vi "main.vi"() -> ()   [LabVIEW 2016]
uses:
  TypeDefs/details.ctl
  TypeDefs/settings.ctl
  TypeDefs/State Enumerate Ring.ctl
  <vilib>/Utility/file.llb/Write Delimited Spreadsheet (DBL).vi
  <instrlib>/Keithley 24XX/Public/Data/Read (Multiple Points).vi
  <instrlib>/Keithley 24XX/Keithley 24XX.lvlib
panel:
  out "Data Output Folder":path
  out "Settings folder path":path
  out "Date array":string[](array[string])
  out "Abort initalisation?":bool
  in  "Tab Control":enum32{"Setup", "Advanced"}(tab)
  in  "Scan settings":T1={"Start voltage (V)"=0.0, "End voltage (V)"=10.0, "Number of steps"=11, "Measurement delay (ms)"=100.0, "Dual sweep"=1, "Stabilisation time (s)"=120.0, "Stabilisation mode"=0, "Stabilisation value (V or A) "=-5.0, "No. of repeat scans"=2.0, "Repeat scans"=0, "Logarithmic sweep"=1, "Electrode configuration"=0} {"Electrode configuration" items=["2-wire", "4-wire"]; "Logarithmic sweep" items=["False", "True"]; "Repeat scans" items=["False", "True"]; "No. of repeat scans" min=1.0 step=1.0; "Stabilisation mode" items=["V", "I"]; "Dual sweep" items=["False", "True"]; "Measurement delay (ms)" min=0.0}
  out "Keithley 2400":bool
  in  "User Name":string
  in  "Exeriment Title":string
  out "Status:":string
  in  "Device details":T2={"Cell Label"="", "Area (cm^2)"=0.0919, "Notes"="", "Scan settings"=0} {"Scan settings" items=["Default", "S01-F-0.1-200-67-0.01-120_-5", "S02-S-0.1-200-67-10-120_-5", "S03-F-0.1-200-67-0.01-0_0", "S04-S-0.1-200-67-10-0_0", "S05-F-0.1-200-67-0.01-10_-5", "S06-F-0.1-200-65-0.01-120_-5", "S07-F-0.001-200-67-0.01-120_-5", "S08-F-0.001-200-67-0.01-120_-10", "S09-F-0.001-200-67-0.01-120_-2", "S12-F-0.1-200-67-0.05-0-0", "S13-F-0.1-200-67-0.01-0-0", "S14-F-0.1-200-67-0.1-0-0", "S15-F-0.01-200-67-0.01-0-0", "S16-F-0.01-20-67-0.01-0-0", "S17-F-0.01-20-67-0.1-0-0", "S18-F-0.1-200-67-0.01-120_-1", "S19-F-0.1-200-67-0.01-120_-1.5", "S20-F-0.1-200-67-0.01-120_-2", "S21-F-0.1-200-67-0.01-120_-2.5", "S22-F-0.1-200-67-0.1-120_-1", "S23-F-0.1-200-67-0.1-120_-2", "S24-F-0.1-200-67-0.1-120_-5", "S25-F-0.1-200-67-0.1-120_-10", "S26-F-0.1-200-67-0.01-120_-10", "S27-F-0.1-200-67-0.01-120_-15", "S28-F-0.1-200-67-0.1-120_-15", "S29-F-0.1-200-67-0.01-12_-5", "S30-F-0.1-200-67-0.01-0-0", "S31-S-0.1-200-67-1-30_-1", "S32-F-0.1-200-200-0.01-120_-1", "S33-F-0.1-200-200-0.01-120_-5", "S34-F-0.1-200-67-0-0_0", "S35-F-0.1-200-67-0-120_-1", "S36-F-0.1-200-67-0-120_-5", "S37-F-0.1-50-67-0.01-0_0", "S38-F-0.1-50-67-0.01-120_1", "S39-F-0.1-100-0.01-120_5", "S40-F-0.1-100-0.002-120-10", "S41-F-0.1-200-0.002-120-10", "S42-F-0.1-200-0.01-120-10", "S43-F-0.1-20-0.01-0_0", "S44-F-0.1-20-67-2-0_0", "S45-F-0.1-80-67-2-0_0", "S46-F-0.1-80-67-2-120_-1"]}
  in  "Delete settings":bool
  in  "Save new settings":bool
  in  "Check Saved Settings":u16(ring) items=["Default", "S01-F-0.1-200-67-0.01-120_-5", "S02-S-0.1-200-67-10-120_-5", "S03-F-0.1-200-67-0.01-0_0", "S04-S-0.1-200-67-10-0_0", "S05-F-0.1-200-67-0.01-10_-5", "S06-F-0.1-200-65-0.01-120_-5", "S07-F-0.001-200-67-0.01-120_-5", "S08-F-0.001-200-67-0.01-120_-10", "S09-F-0.001-200-67-0.01-120_-2", "S12-F-0.1-200-67-0.05-0-0", "S13-F-0.1-200-67-0.01-0-0", "S14-F-0.1-200-67-0.1-0-0", "S15-F-0.01-200-67-0.01-0-0", "S16-F-0.01-20-67-0.01-0-0", "S17-F-0.01-20-67-0.1-0-0", "S18-F-0.1-200-67-0.01-120_-1", "S19-F-0.1-200-67-0.01-120_-1.5", "S20-F-0.1-200-67-0.01-120_-2", "S21-F-0.1-200-67-0.01-120_-2.5", "S22-F-0.1-200-67-0.1-120_-1", "S23-F-0.1-200-67-0.1-120_-2", "S24-F-0.1-200-67-0.1-120_-5", "S25-F-0.1-200-67-0.1-120_-10", "S26-F-0.1-200-67-0.01-120_-10", "S27-F-0.1-200-67-0.01-120_-15", "S28-F-0.1-200-67-0.1-120_-15", "S29-F-0.1-200-67-0.01-12_-5", "S30-F-0.1-200-67-0.01-0-0", "S31-S-0.1-200-67-1-30_-1", "S32-F-0.1-200-200-0.01-120_-1", "S33-F-0.1-200-200-0.01-120_-5", "S34-F-0.1-200-67-0-0_0", "S35-F-0.1-200-67-0-120_-1", "S36-F-0.1-200-67-0-120_-5", "S37-F-0.1-50-67-0.01-0_0", "S38-F-0.1-50-67-0.01-120_1", "S39-F-0.1-100-0.01-120_5", "S40-F-0.1-100-0.002-120-10", "S41-F-0.1-200-0.002-120-10", "S42-F-0.1-200-0.01-120-10", "S43-F-0.1-20-0.01-0_0", "S44-F-0.1-20-67-2-0_0", "S45-F-0.1-80-67-2-0_0", "S46-F-0.1-80-67-2-120_-1"]
  in  "Save New Settings As...":string
  in  "Update":bool
  in  "Exit":bool
  out "JV Curve":cluster{dbl[], dbl[]}(graph)
  in  "Start Scan":bool
  in  "error in (no error) 3":errorcluster
  in  "VISA resource name":refnum<visa-resource-name>="GPIB1::26::INSTR"
  # "Connected instruments"
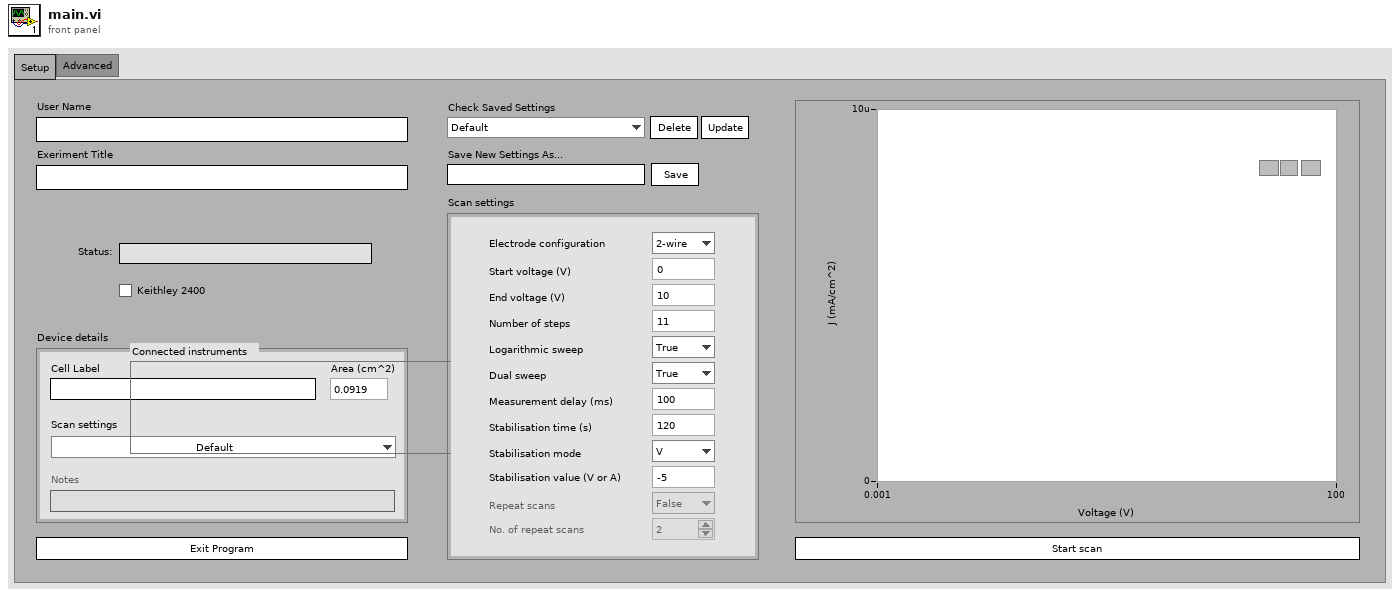
[diagram p1: front panel]
types:
  T1 = typedef "settings.ctl" = cluster{"Start voltage (V)":dbl, "End voltage (V)":dbl, "Number of steps":u32, "Measurement delay (ms)":dbl, "Dual sweep":u16, "Stabilisation time (s)":dbl, "Stabilisation mode":u16, "Stabilisation value (V or A) ":dbl, "No. of repeat scans":dbl, "Repeat scans":u16, "Logarithmic sweep":u16, "Electrode configuration":u16}
  T2 = typedef "details.ctl" = cluster{"Cell Label":string, "Area (cm^2)":dbl, "Notes":string, "Scan settings":u16}
  T3 = typedef "State Enumerate Ring.ctl" = enum16{"Initialise", "Idle", "Measure", "Notify"}
  T4 = enum8{"Enabled", "Disabled", "Disabled and Grayed Out"}
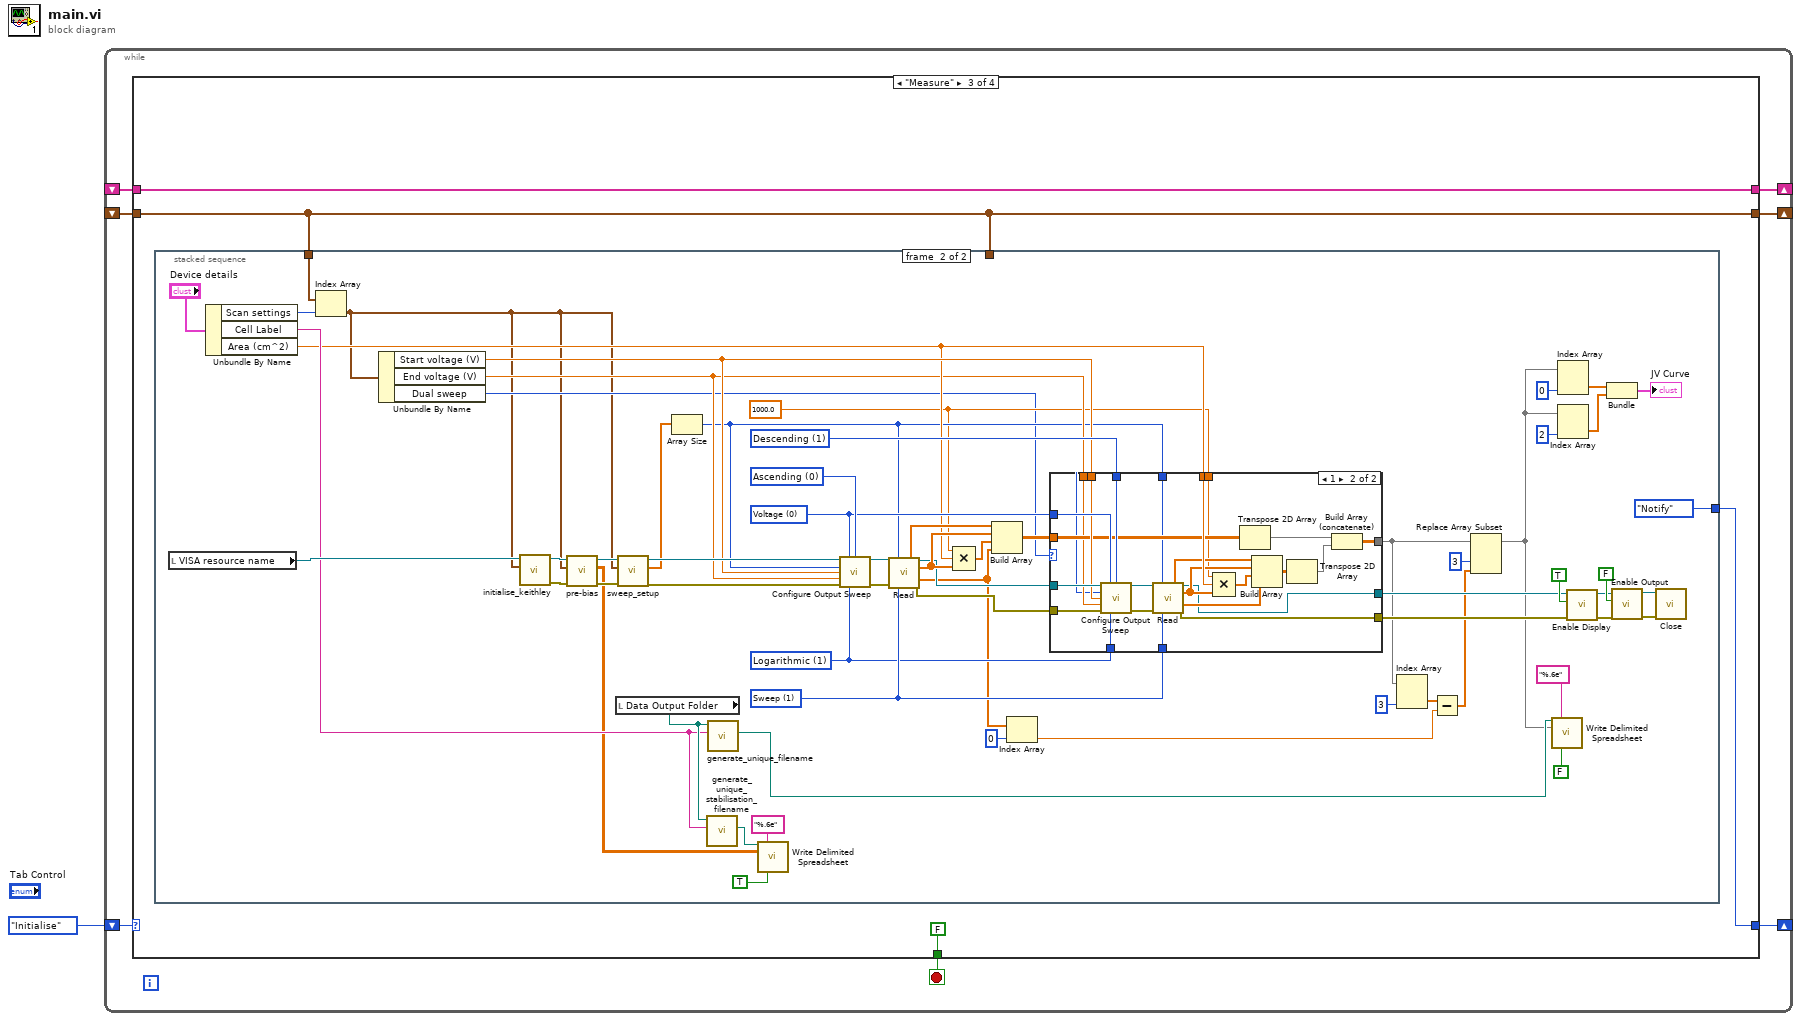
[diagram p0: block diagram]
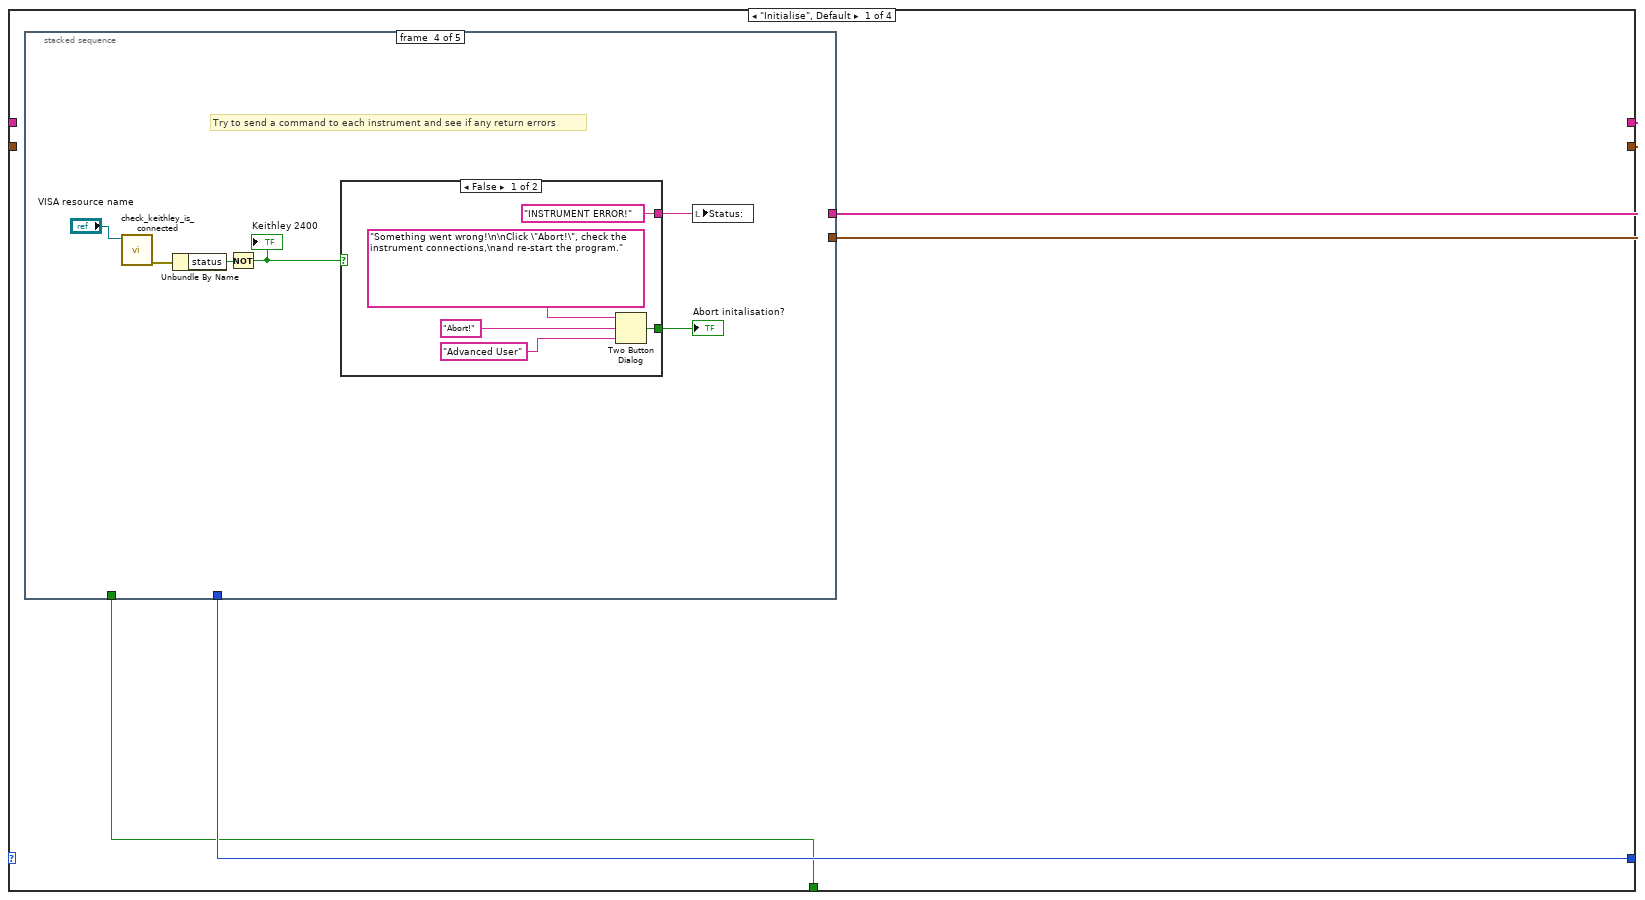
[diagram p2: hidden frame]
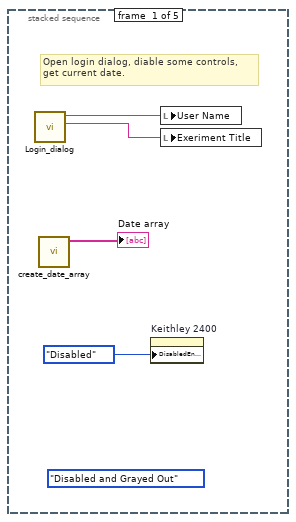
[diagram p3: hidden frame]
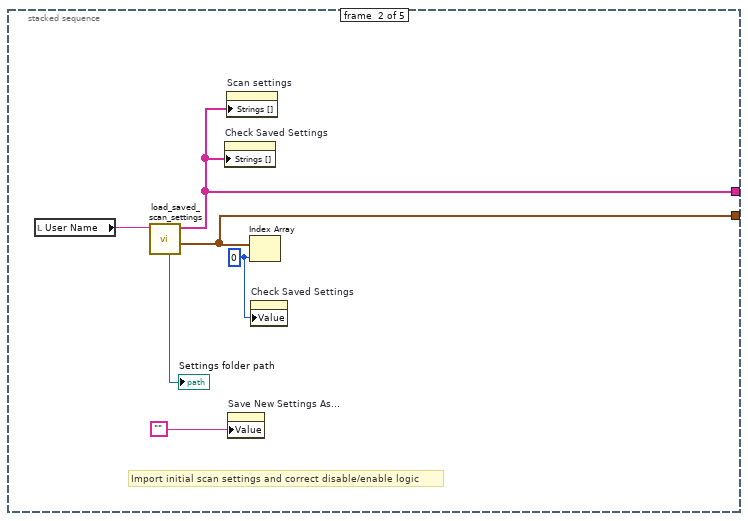
[diagram p4: hidden frame]
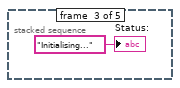
[diagram p5: hidden frame]
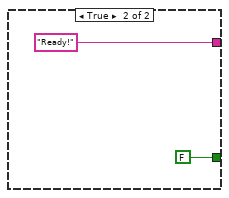
[diagram p6: hidden frame]
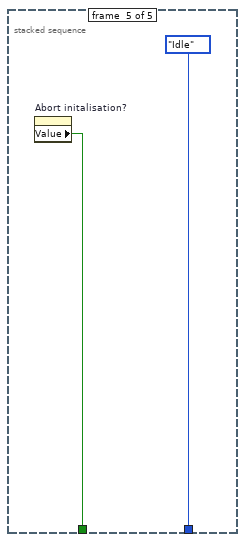
[diagram p7: hidden frame]
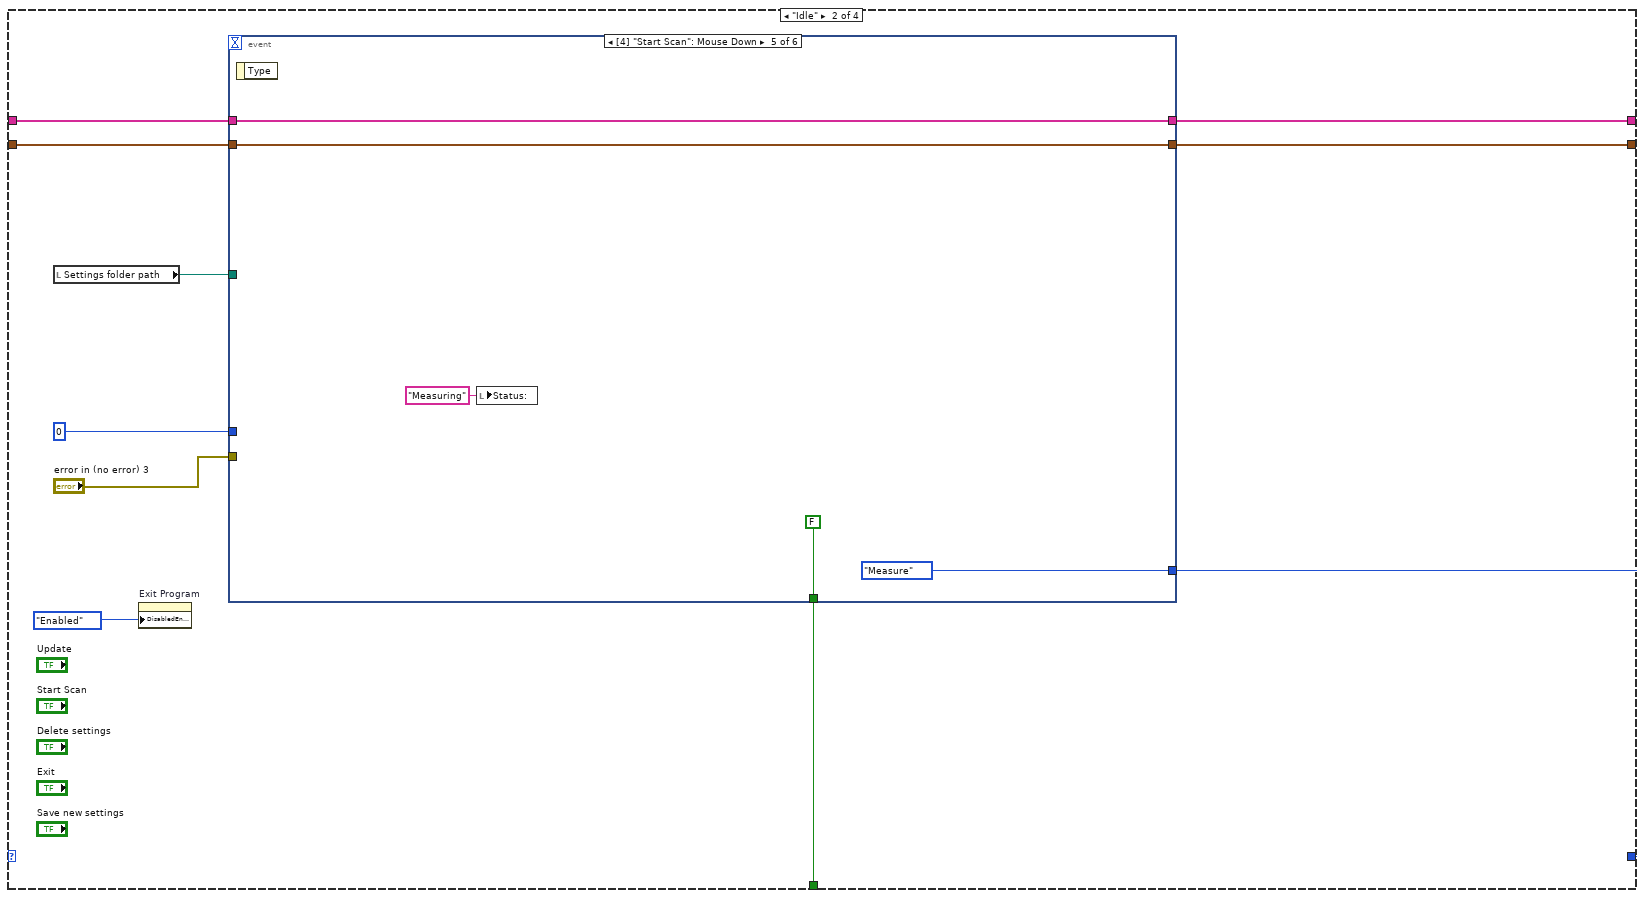
[diagram p8: hidden frame]
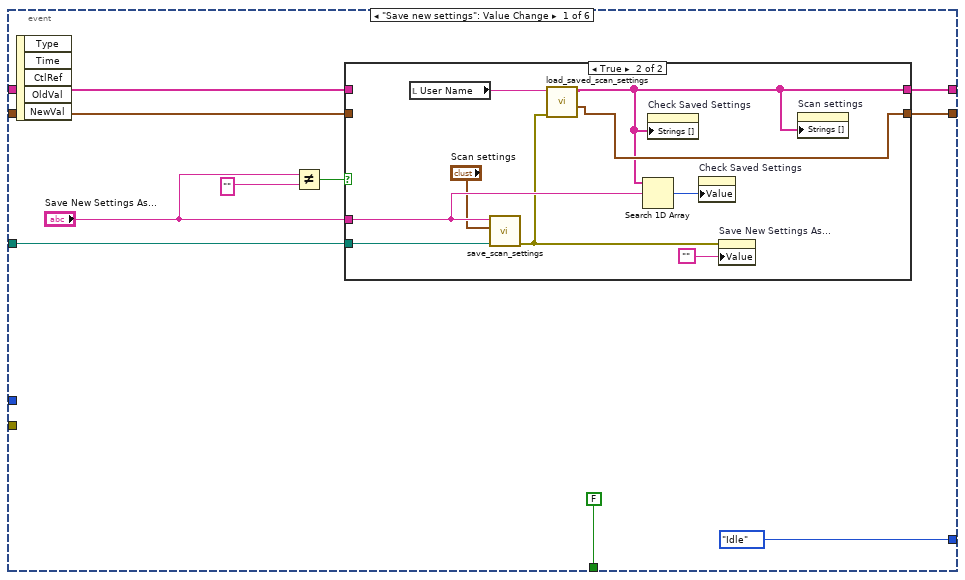
[diagram p9: hidden frame]
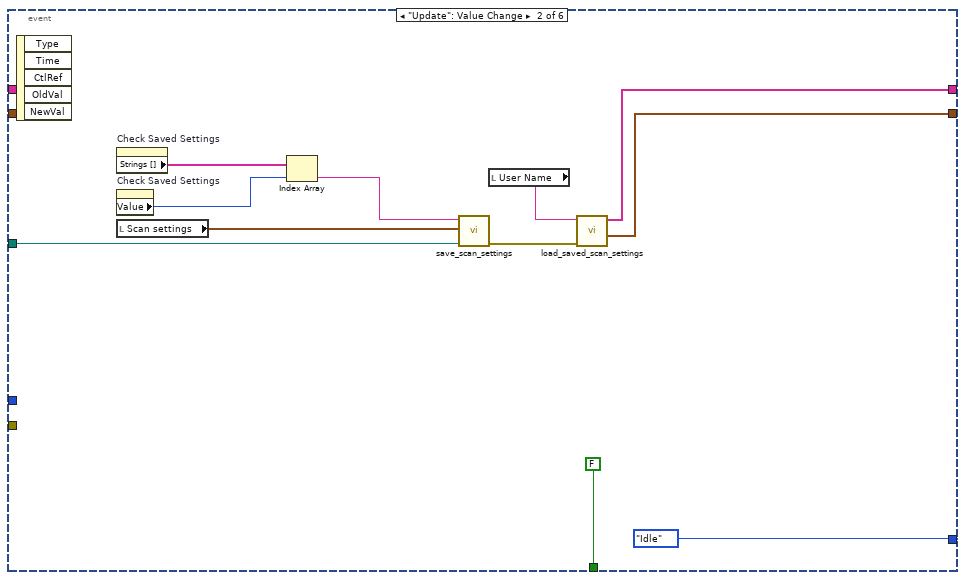
[diagram p11: hidden frame]
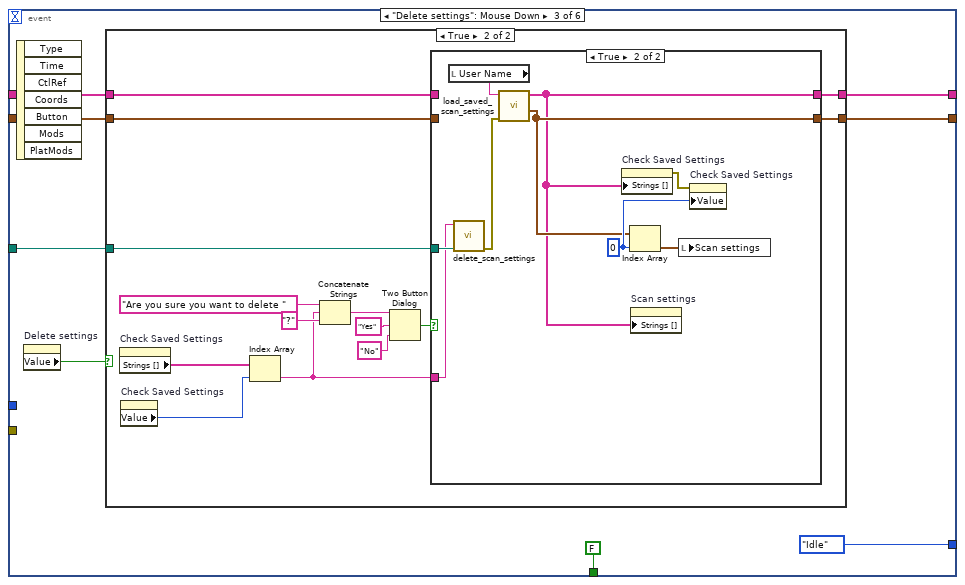
[diagram p12: hidden frame]
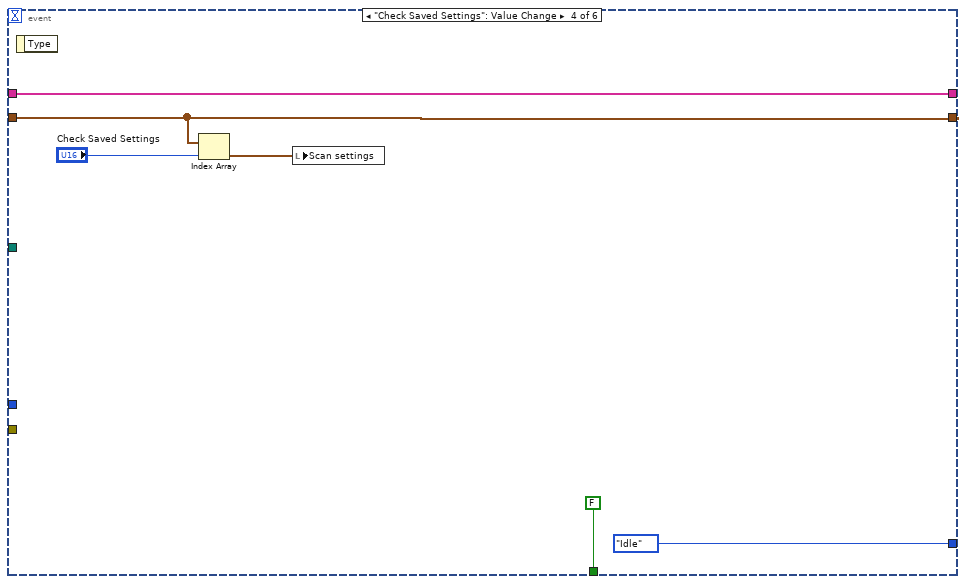
[diagram p15: hidden frame]
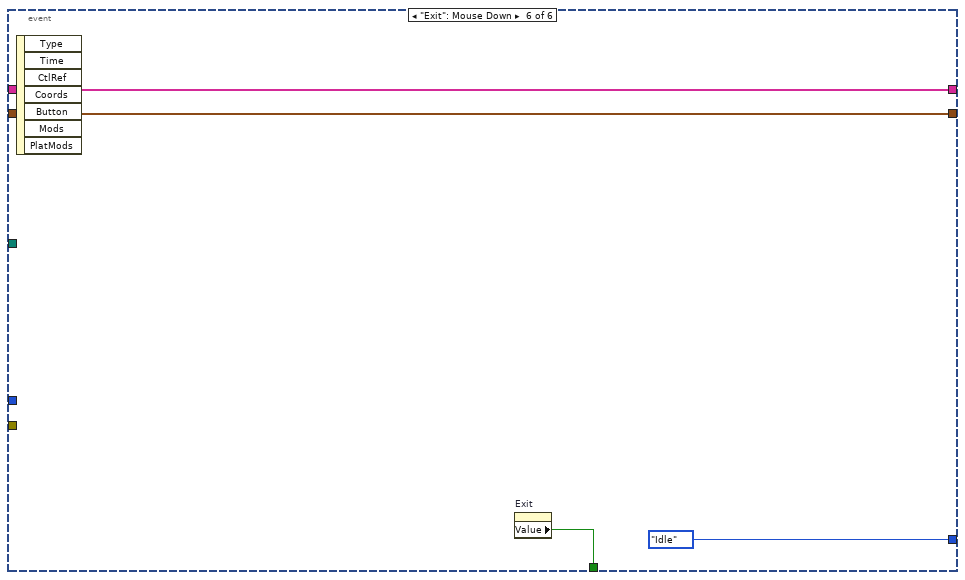
[diagram p16: hidden frame]
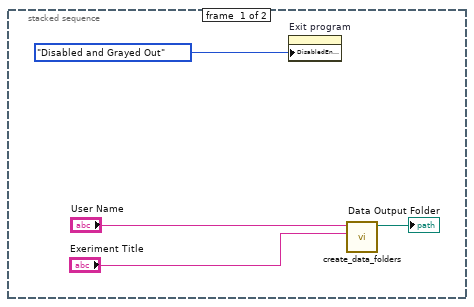
[diagram p17: hidden frame]
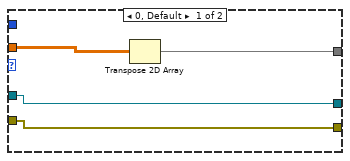
[diagram p18: hidden frame]
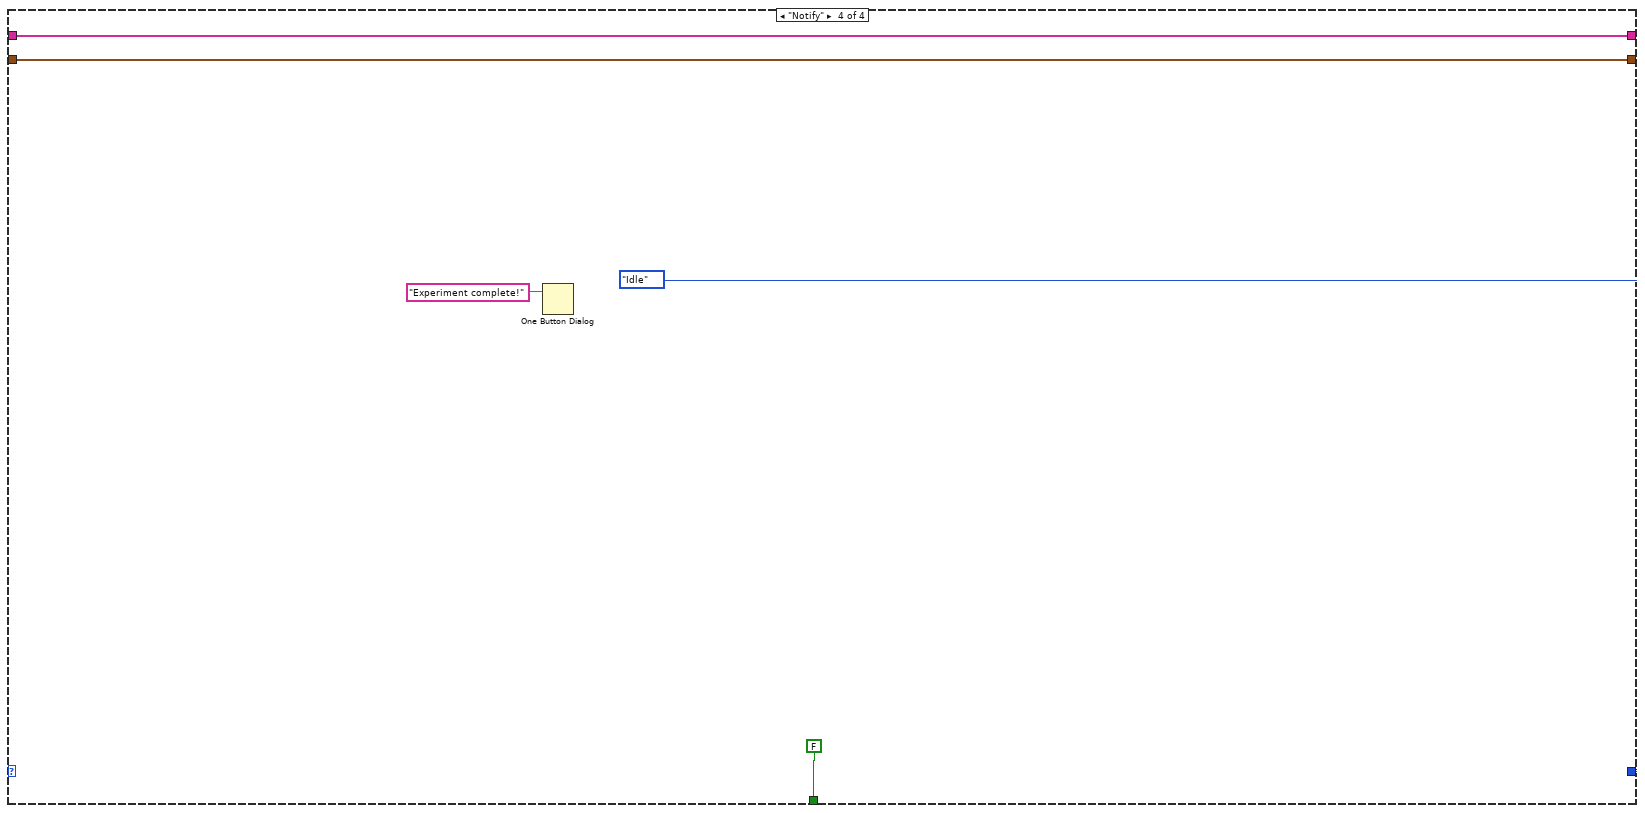
[diagram p19: hidden frame]
diagram:
  n1 = while {
    shift-right: [w3] -> _
    shift-left: _ -> [w5]
    shift-right: [w4] -> _
    shift-left: _ -> [w6]
    shift-right: [w7] -> _
    shift-left: State_Enumerate_Ring."Initialise" ("Enum") -> [w8]
    stop <- w2 stop-if-true
    n2 = case shown="\"Measure\"" w8 {
      tunnel: [w12 w42 w132 State_Enumerate_Ring."Idle" ("Enum")] -> w7
      tunnel: w6 -> [_ w46 w131 w234]
      tunnel: w5 -> [_ w45 w133 w233]
      tunnel: [w10 w44 w131 w234] -> w4
      tunnel: [w9 w43 w133 w233] -> w3
      tunnel: [w11 w40 FALSE ("Value") FALSE ("Value")] -> w2
      frame "Initialise", Default {
        n3 = stacked-sequence {
          tunnel: [_ _ _ _ State_Enumerate_Ring."Idle" ("Enum")] -> w12
          tunnel: [_ _ _ _ w37] -> w11
          tunnel: [_ w22 _ _ _] -> w10
          tunnel: [_ w21 _ _ _] -> w9
          frame #0 {
            (unwired) T4."Disabled and Grayed Out" ("Disabled")
            # "Open login dialog, diable some controls,\nget current date."
            n4 = call "Login_dialog.vi"() -> ("Experiment title out"=w13:string, "User name out"=w14:string)  [unwired: 10 in]
            n5 = call "create_date_array.vi"() -> ("Date Array"=→"Date array":string[])  [unwired: 11 in]
            n6 = property on="Keithley 2400" class="Bool (strict)"("DisabledEnum"=T4."Disabled" ("Disabled")) -> ()  [unwired: 2 in, 2 out]
            n7 = local write "User Name"(w14) -> ()
            n8 = local write "Exeriment Title"(w13) -> ()
          }
          frame #1 {
            w19 = 0 ("index")
            # "Import initial scan settings and correct disable/enable logic"
            n9 = local read "User Name"() -> (w17:string)
            n10 = call "load_saved_scan_settings.vi"("User name"=w17) -> ("Scan settings array"=w21:T1[], "Scan settings name array"=w22:string[], "Settings folder path"=→"Settings folder path":path)  [unwired: 7 in, 1 out]
            n11 = property on="Check Saved Settings" class="Ring (strict)"("Strings []"=w22) -> ()  [unwired: 2 in, 2 out]
            n12 = property on="Scan settings" class="Ring (strict)"("Strings []"=w22) -> ()  [unwired: 2 in, 2 out]
            n13 = property on="Save New Settings As..." class="Str"("Value"="") -> ()  [unwired: 2 in, 2 out]
            n14 = Index Array(array=w21, index=w19) -> ()  [unwired: 1 out]
            n15 = property on="Check Saved Settings" class="Ring (strict)"("Value"=w19) -> ()  [unwired: 2 in, 2 out]
          }
          frame #2 {
            "Status:" <- "Initialising..." ("Instrument status")
          }
          frame #3 {
            # "Try to send a command to each instrument and see if any return errors"
            n16 = call "check_keithley_is_connected.vi"("VISA resource name"="VISA resource name") -> ("error out"=w29:errorcluster)  [unwired: 10 in]
            n17 = Unbundle By Name(w29) -> ("status"=w27:bool)
            n18 = Not(x=w27) -> (.not. x?=w25:bool)
            "Keithley 2400" <- w25
            n19 = case shown="False" w25 {
              tunnel: ["INSTRUMENT ERROR!" ("Instrument status") "Ready!" ("Instrument status")] -> w28
              tunnel: [w32 FALSE ("T button?")] -> w26
              frame False {
                n20 = Two Button Dialog(message="Something went wrong!\n\nClick \"Abort!\", check the instrument connections,\nand re-start the program.", 1:"Advanced User" ("T button name (\"OK\")"), 2:"Abort!" ("F button name (\"Cancel\")")) -> (T button?=w32:bool)
              }
              frame True {
              }
            }
            "Abort initalisation?" <- w26
            n21 = local write "Status:"(w28) -> ()
          }
          frame #4 {
            n22 = property on="Abort initalisation?" class="Bool (strict)"() -> ("Value"=w37:bool)  [unwired: 2 in, 2 out]
          }
        }
      }
      frame "Idle" {
        n23 = local read "Settings folder path"() -> (w39:path)
        n24 = property on="Exit Program" class="Bool (strict)"("DisabledEnum"=T4."Enabled" ("Disabled")) -> ()  [unwired: 2 in, 2 out]
        n25 = event shown="[4] \"Start Scan\": Mouse Down" {
          selector: _ -> [_ _ _ _ _ _]
          dyn-events: _ -> [_ _ _ _ _ _]
          timeout: _ -> [_ _ _ _ _ _]
          tunnel: 0 -> [_ _ _ _ _ _]
          tunnel: "error in (no error) 3" -> [_ _ _ _ _ _]
          tunnel: w46 -> [w52 _ w87 w120 w125 w130]
          tunnel: w45 -> [w51 _ w88 w119 w124 w129]
          tunnel: w39 -> [w56 w77 w84 _ _ _]
          tunnel: [w55 w73 w86 w120 w125 w130] -> w44
          tunnel: [w54 w72 w85 w119 w124 w129] -> w43
          tunnel: [State_Enumerate_Ring."Idle" ("Enum") State_Enumerate_Ring."Idle" ("Enum") State_Enumerate_Ring."Idle" ("Enum") State_Enumerate_Ring."Idle" ("Enum") State_Enumerate_Ring."Measure" ("Enum") State_Enumerate_Ring."Idle" ("Enum")] -> w42
          tunnel: [FALSE ("Value") FALSE ("Value") FALSE ("Value") FALSE ("Value") FALSE ("Value") w127] -> w40
          event "Save new settings": Value Change {
            n26 = event-data() -> ()  [unwired: 1 in, 5 out]
            n27 = Not Equal?(x="Save New Settings As...", y="") -> (x != y?=w49:bool)
            n28 = case shown="True" w49 {
              tunnel: [w59 w68] -> w54
              tunnel: [w60 w62] -> w55
              tunnel: w56 -> [_ w69]
              tunnel: "Save New Settings As..." -> [_ w67]
              tunnel: w52 -> [w60 _]
              tunnel: w51 -> [w59 _]
              frame False {
              }
              frame True {
                n29 = local read "User Name"() -> (w63:string)
                n30 = call "save_scan_settings.vi"("Path"=w69, "New scan settings"="Scan settings", "New name"=w67) -> ("error out"=w64:errorcluster)  [unwired: 8 in]
                n31 = call "load_saved_scan_settings.vi"("error in (no error)"=w64, "User name"=w63) -> ("Scan settings array"=w68:T1[], "Scan settings name array"=w62:string[])  [unwired: 6 in, 2 out]
                n32 = Search 1D Array(1D array=w62, element=w67) -> (index of element=w66:i32)  [unwired: 1 in]
                n33 = property on="Check Saved Settings" class="Ring (strict)"("Strings []"=w62) -> ()  [unwired: 2 in, 2 out]
                n34 = property on="Check Saved Settings" class="Ring (strict)"("Value"=w66) -> ()  [unwired: 2 in, 2 out]
                n35 = property on="Save New Settings As..." class="Str"(error in=w64, "Value"="") -> ()  [unwired: 1 in, 2 out]
                n36 = property on="Scan settings" class="Ring (strict)"("Strings []"=w62) -> ()  [unwired: 2 in, 2 out]
              }
            }
          }
          event "Update": Value Change {
            n37 = event-data() -> ()  [unwired: 1 in, 5 out]
            n38 = property on="Check Saved Settings" class="Ring (strict)"() -> ("Strings []"=w80:string[])  [unwired: 2 in, 2 out]
            n39 = property on="Check Saved Settings" class="Ring (strict)"() -> ("Value"=w79:u16)  [unwired: 2 in, 2 out]
            n40 = local read "Scan settings"() -> (w70:T1)
            n41 = Index Array(array=w80, index=w79) -> (element=w78:string)
            n42 = call "save_scan_settings.vi"("Path"=w77, "New scan settings"=w70, "New name"=w78) -> ("error out"=w74:errorcluster)  [unwired: 8 in]
            n43 = local read "User Name"() -> (w71:string)
            n44 = call "load_saved_scan_settings.vi"("error in (no error)"=w74, "User name"=w71) -> ("Scan settings array"=w72:T1[], "Scan settings name array"=w73:string[])  [unwired: 6 in, 2 out]
          }
          event "Delete settings": Mouse Down {
            n45 = event-data() -> ()  [unwired: 1 in, 7 out]
            n46 = property on="Delete settings" class="Bool (strict)"() -> ("Value"=w83:bool)  [unwired: 2 in, 2 out]
            n47 = case shown="True" w83 {
              tunnel: w88 -> [w89 w96]
              tunnel: w87 -> [w90 w95]
              tunnel: [w90 w94] -> w86
              tunnel: [w89 w93] -> w85
              tunnel: w84 -> [_ w92]
              frame False {
              }
              frame True {
                n48 = property on="Check Saved Settings" class="Ring (strict)"() -> ("Strings []"=w102:string[])  [unwired: 2 in, 2 out]
                n49 = property on="Check Saved Settings" class="Ring (strict)"() -> ("Value"=w101:u16)  [unwired: 2 in, 2 out]
                n50 = Index Array(array=w102, index=w101) -> (element=w91:string)
                n51 = Concatenate Strings("Are you sure you want to delete " ("string"), w91, "?" ("string")) -> (w98:string)
                n52 = Two Button Dialog(message=w98, 1:"No" ("F button name (\"Cancel\")"), 2:"Yes" ("T button name (\"OK\")")) -> (T button?=w97:bool)
                n53 = case shown="True" w97 {
                  tunnel: w96 -> [w105 _]
                  tunnel: w95 -> [w106 _]
                  tunnel: [w106 w108] -> w94
                  tunnel: [w105 w111] -> w93
                  tunnel: w92 -> [_ w115]
                  tunnel: w91 -> [_ w114]
                  frame False {
                  }
                  frame True {
                    w113 = 0 ("index")
                    n54 = local read "User Name"() -> (w109:string)
                    n55 = call "delete_scan_settings.vi"("Path"=w115, "Scan settings name"=w114) -> ("error out"=w110:errorcluster)  [unwired: 9 in]
                    n56 = call "load_saved_scan_settings.vi"("error in (no error)"=w110, "User name"=w109) -> ("Scan settings array"=w111:T1[], "Scan settings name array"=w108:string[])  [unwired: 6 in, 2 out]
                    n57 = property on="Check Saved Settings" class="Ring (strict)"("Strings []"=w108) -> (error out=w112:errorcluster)  [unwired: 2 in, 1 out]
                    n58 = Index Array(array=w111, index=w113) -> (element=w107:T1)
                    n59 = property on="Scan settings" class="Ring (strict)"("Strings []"=w108) -> ()  [unwired: 2 in, 2 out]
                    n60 = local write "Scan settings"(w107) -> ()
                    n61 = property on="Check Saved Settings" class="Ring (strict)"(error in=w112, "Value"=w113) -> ()  [unwired: 1 in, 2 out]
                  }
                }
              }
            }
          }
          event "Check Saved Settings": Value Change {
            n62 = event-data() -> ()  [unwired: 1 in, 1 out]
            n63 = Index Array(array=w119, index="Check Saved Settings") -> (element=w116:T1)
            n64 = local write "Scan settings"(w116) -> ()
          }
          event "Start Scan": Mouse Down {
            n65 = event-data() -> ()  [unwired: 1 in, 1 out]
            n66 = local write "Status:"("Measuring" ("Status:")) -> ()
          }
          event "Exit": Mouse Down {
            n67 = event-data() -> ()  [unwired: 1 in, 7 out]
            n68 = property on="Exit" class="Bool (strict)"() -> ("Value"=w127:bool)  [unwired: 2 in, 2 out]
          }
        }
      }
      frame "Measure" {
        n69 = stacked-sequence {
          tunnel: w133 -> [_ _]
          tunnel: [_ State_Enumerate_Ring."Notify" ("Enum")] -> w132
          tunnel: w133 -> [_ w195]
          frame #0 {
            n70 = property on="Exit program" class="Bool (strict)"("DisabledEnum"=T4."Disabled and Grayed Out" ("Disabled")) -> ()  [unwired: 2 in, 2 out]
            n71 = call "create_data_folders.vi"("Experiment Indicator"="Exeriment Title", "username"="User Name") -> ("Data Output Folder"=→"Data Output Folder":path)  [unwired: 9 in]
          }
          frame #1 {
            w150 = 1000.0 ("value")
            w164 = u16 1 items=["Ascending", "Descending"] ("Sweep Direction  (0: Ascending)")
            w169 = u16 0 items=["Ascending", "Descending"] ("Sweep Direction  (0: Ascending)")
            w159 = u16 1 items=["Linear", "Logarithmic"] ("Sweep Spacing  (0: Linear)")
            w161 = u16 1 items=["Fixed", "Sweep", "List"] ("Output Mode (0: Fixed)")
            w163 = u16 0 items=["Voltage", "Current"] ("Source Mode  (0: Voltage)")
            n72 = local read "VISA resource name"() -> (w200:refnum<visa-resource-name>)
            n73 = Unbundle By Name("Device details") -> ("Scan settings"=w196:u16, "Cell Label"=w191:string, "Area (cm^2)"=w160:dbl)
            n74 = Index Array(array=w195, index=w196) -> (element=w139:T1)
            n75 = Unbundle By Name(w139) -> ("Start voltage (V)"=w162:dbl, "End voltage (V)"=w152:dbl, "Dual sweep"=w149:u16)
            n76 = call "initialise_keithley.vi"("Scan settings"=w139, "VISA Refnum in"=w200) -> ("error out"=w198:errorcluster, "VISA Refnum out"=w199:refnum<visa-resource-name>)  [unwired: 8 in]
            n77 = call "pre-bias.vi"("error in (no error)"=w198, "Check scan settings"=w139, "VISA resource name in"=w199) -> ("error out"=w193:errorcluster, "Stabilisation data"=w189:dbl[][], "VISA resource name out"=w194:refnum<visa-resource-name>)  [unwired: 5 in]
            n78 = local read "Data Output Folder"() -> (w192:path)
            n79 = call "sweep_setup.vi"("error in (no error)"=w193, "Check scan settings"=w139, "VISA Refnum in"=w194) -> ("error out"=w176:errorcluster, "Voltage list"=w173:dbl[], "VISA Refnum out"=w177:refnum<visa-resource-name>)  [unwired: 6 in]
            n80 = Array Size(array=w173) -> (size(s)=w151:i32)
            n81 = call "generate_unique_stabilisation_filename.vi"("Filename (no extension)"=w191, "Data Folder"=w192) -> ("Filename"=w190:path)  [unwired: 9 in]
            n82 = call "generate_unique_filename.vi"("Filename (no extension)"=w191, "Data Folder"=w192) -> ("Filename"=w182:path)  [unwired: 9 in]
            n83 = call-poly <vilib>:"Write Delimited Spreadsheet.vi"("file path (dialog if empty)"=w190, "format (%.3f)"="%.6e", "2D data"=w189, "transpose? (no:F)"=TRUE) -> ()  [unwired: 10 in, 2 out]
            n84 = call <instrlib>:"Configure Output Sweep.vi"("VISA resource name"=w177, "Source Mode  (0: Voltage)"=w163, "Sweep Direction  (0: Ascending)"=w169, "Number of Points (5)"=w151, "Minimum Amplitude (1)"=w162, "Maximum Amplitude (2)"=w152, "error in (no error)"=w176, "Sweep Spacing  (0: Linear)"=w159) -> ("VISA resource name out"=w175:refnum<visa-resource-name>, "error out"=w174:errorcluster)  [unwired: 6 in]
            n85 = call-poly <instrlib>:"Read.vi"("VISA resource name"=w175, "Sample Count (1)"=w151, "error in (no error)"=w174, "Output Mode (0: Fixed)"=w161) -> ("Voltage"=w180:sgl[], "VISA resource name out"=w166:refnum<visa-resource-name>, "Current"=w179:sgl[], "Timestamp"=w148:sgl[], "error out"=w165:errorcluster)  [unwired: 5 in, 2 out]
            n86 = Compound Arithmetic op=MULTIPLY(w150, w160, w179) -> (w178:dbl[])
            n87 = Build Array(w180, w179, w178, w148) -> (w158:dbl[][])
            n88 = Index Array(array=w148, index=0) -> (element=w144:sgl)
            n89 = case shown="1" w149 {
              tunnel: w166 -> [w204 w229]
              tunnel: w165 -> [w205 w228]
              tunnel: w164 -> [_ w227]
              tunnel: w163 -> [_ w226]
              tunnel: w162 -> [_ w225]
              tunnel: w161 -> [_ w222]
              tunnel: w160 -> [_ w221]
              tunnel: w159 -> [_ w216]
              tunnel: w158 -> [w203 w215]
              tunnel: [w202 w211] -> w143
              tunnel: [w204 w210] -> w156
              tunnel: [w205 w209] -> w155
              tunnel: w152 -> [_ w208]
              tunnel: w151 -> [_ w207]
              tunnel: w150 -> [_ w206]
              frame 0, Default {
                n90 = Transpose 2D Array(2D array=w203) -> (transposed array=w202:dbl[][])
              }
              frame 1 {
                n91 = call <instrlib>:"Configure Output Sweep.vi"("VISA resource name"=w229, "Source Mode  (0: Voltage)"=w226, "Sweep Direction  (0: Ascending)"=w227, "Number of Points (5)"=w207, "Minimum Amplitude (1)"=w225, "Maximum Amplitude (2)"=w208, "error in (no error)"=w228, "Sweep Spacing  (0: Linear)"=w216) -> ("VISA resource name out"=w224:refnum<visa-resource-name>, "error out"=w223:errorcluster)  [unwired: 6 in]
                n92 = call-poly <instrlib>:"Read.vi"("VISA resource name"=w224, "Sample Count (1)"=w207, "error in (no error)"=w223, "Output Mode (0: Fixed)"=w222) -> ("Voltage"=w219:sgl[], "VISA resource name out"=w210:refnum<visa-resource-name>, "Current"=w218:sgl[], "Timestamp"=w217:sgl[], "error out"=w209:errorcluster)  [unwired: 5 in, 2 out]
                n93 = Compound Arithmetic op=MULTIPLY(w206, w221, w218) -> (w220:dbl[])
                n94 = Transpose 2D Array(2D array=w215) -> (transposed array=w213:dbl[][])
                n95 = Build Array(w219, w218, w220, w217) -> (w214:dbl[][])
                n96 = Transpose 2D Array(2D array=w214) -> (transposed array=w212:dbl[][])
                n97 = Build Array (concatenate)(w213, w212) -> (w211:dbl[][])
              }
            }
            n98 = Index Array(array=w143, index (col)=3 ("disabled index (col)")) -> (element=w145:dbl[])  [unwired: 1 in]
            n99 = Subtract(x=w145, y=w144) -> (x-y=w141:dbl[])
            n100 = Replace Array Subset(array=w143, new element=w141, index (col)=3 ("disabled index (col)")) -> (w140:dbl[][])  [unwired: 1 in]
            n101 = call-poly <vilib>:"Write Delimited Spreadsheet.vi"("file path (dialog if empty)"=w182, "format (%.3f)"="%.6e", "2D data"=w140, "transpose? (no:F)"=FALSE) -> ()  [unwired: 10 in, 2 out]
            n102 = Index Array(array=w140, index (col)=0 ("disabled index (col)")) -> (element=w185:dbl[])  [unwired: 1 in]
            n103 = Index Array(array=w140, index (col)=2 ("disabled index (col)")) -> (element=w186:dbl[])  [unwired: 1 in]
            n104 = call <instrlib>:"Enable Display.vi"("error in (no error)"=w155, "Enable Display (T: Enable)"=TRUE, "VISA resource name"=w156) -> ("error out"=w154:errorcluster, "VISA resource name out"=w153:refnum<visa-resource-name>)  [unwired: 7 in]
            n105 = Bundle(w185, w186) -> (→"JV Curve":cluster{dbl[], dbl[]})  [unwired: 1 in]
            n106 = call <instrlib>:"Enable Output.vi"("error in (no error)"=w154, "Enable Output (T: Enable)"=FALSE ("Output (Off)"), "VISA resource name"=w153) -> ("error out"=w170:errorcluster, "VISA resource name out"=w171:refnum<visa-resource-name>)  [unwired: 7 in]
            n107 = call <instrlib>:"Close.vi"("error in (no error)"=w170, "VISA resource name"=w171) -> ()  [unwired: 9 in, 1 out]
          }
        }
      }
      frame "Notify" {
        n108 = One Button Dialog(message="Experiment complete!") -> ()  [unwired: 1 in, 1 out]
      }
    }
  }
